vi "Launch Mission Actor.vi"(11 "RDS Root Actor in":refnum<class "RDS Root Actor.lvclass">) -> (3 "RDS Root Actor out":refnum<class "RDS Root Actor.lvclass">)   [LabVIEW 2015, in "RDS Root Actor.lvlib" / "RDS Root Actor.lvclass"]
uses:
  RDS Root Actor.lvclass
  Libraries/RDS Framework/RDS Message ID.ctl
  RDS Mission Controller Actor/RDS Mission Controller Actor/RDS Mission Controller Actor.lvclass
  RDS Mission Controller Actor/RDS Mission Controller Actor/RDS Mission Controller Actor.lvclass/RDS Mission Controller Actor.ctl
  RDS Parent Actor/RDS Parent Actor/RDS Parent Actor.lvclass/RDS Parent Actor.ctl
  RDS Parent Actor/RDS Parent Actor/RDS Parent Actor.lvclass
  Libraries/RDS Child Messages/RDS Child Messages.lvlib
  Libraries/Configuration Library/RDS Configuration Library.lvlib
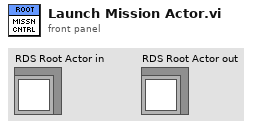
[diagram p1: front panel]
types:
  T1 = typedef "RDS Child Messages.lvlib/RDS Message ID.ctl" = enum16{"RDS Hello World", "String Message", "AIP_Status", "AIP_Command", "GPS_Data", "MCB_Command", "MCB_Status", "Compass_Data", "Depth_Data", "Battery_Data", "Contoller_State", "Set_Mag_Dev", "BTB_Shutdown", "State_Sample_Request", "State_Sample", "PID_Gains_Set", "Helm_Limiter_Set", "Helm_Heading_Command", "Helm_Steering_Command", "Helm_Status", "Controller_Message", "AIP_Set_Min_Depth", "Mission_Controller_State", "Mission_Upload", "Mission_Set_Op_and_Run", "Mission_Settings_Set"}
  T2 = typedef "RDS Configuration Library.lvlib/RDS Configuration.ctl" = cluster{"State Update Rate (Hz)":dbl, "Helm Rate (Hz)":dbl, "Helm Gains":T3, "Limiter":dbl, "Mission Controller Settings":T4, "Mag Dev":dbl}
  T3 = typedef "RDS Child Messages.lvlib/PID Gains Control.ctl" = cluster{"P (Kc)":sgl, "I (Ti)":sgl, "D (Td)":sgl}
  T4 = typedef "RDS Mission Controller Actor.lvlib/Mission Controller Settings.ctl" = cluster{"Waypoint Radius (m)":dbl}
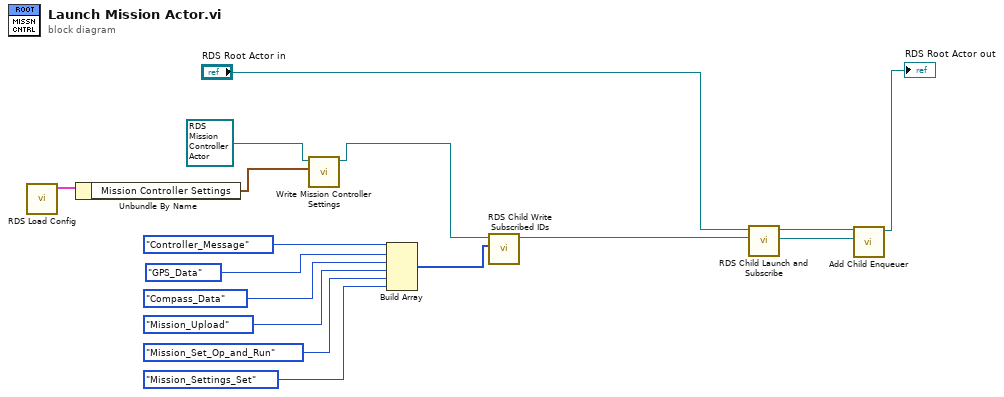
[diagram p0: block diagram]
diagram:
  n1 = call "RDS Load Config.vi"() -> ("RDS Config"=w7:T2)  [unwired: 11 in]
  n2 = Unbundle By Name(w7) -> ("Mission Controller Settings"=w6:T4)
  n3 = call "Write Mission Controller Settings.vi"("Mission Controller Settings"=w6, "RDS Mission Controller Actor in"=refnum<class "RDS Mission Controller Actor.lvclass"> refnum ("RDS Mission Controller Actor.lvlib:RDS Mission Controller Actor.lvclass")) -> ("RDS Mission Controller Actor out"=w8:refnum<class "RDS Mission Controller Actor.lvclass">)  [unwired: 8 in, 1 out]
  n4 = Build Array(RDS_Message_ID."Controller_Message" ("RDS Message"), RDS_Message_ID."GPS_Data" ("RDS Message"), RDS_Message_ID."Compass_Data" ("RDS Message"), RDS_Message_ID."Mission_Upload" ("RDS Message"), RDS_Message_ID."Mission_Set_Op_and_Run" ("RDS Message"), RDS_Message_ID."Mission_Settings_Set" ("RDS Message")) -> (w10:T1[])
  n5 = call "RDS Child Write Subscribed IDs.vi"("Subscribed IDs"=w10, "RDS Parent Actor in"=w8) -> ("RDS Parent Actor out"=w13:refnum<class "RDS Mission Controller Actor.lvclass">)  [unwired: 8 in, 1 out]
  n6 = call "RDS Child Launch and Subscribe.vi"("RDS Child in"=w13, "Caller Actor in"="RDS Root Actor in") -> ("Nested Actor's Enqueuer"=w15:refnum<class "Message Enqueuer.lvclass">, "Caller Actor Out"=w14:refnum<class "RDS Root Actor.lvclass">)  [unwired: 7 in, 1 out]
  n7 = call "Add Child Enqueuer.vi"("Nested Actor's Enqueuer"=w15, "RDS Root Actor in"=w14) -> ("RDS Root Actor out"=→"RDS Root Actor out":refnum<class "RDS Root Actor.lvclass">)  [unwired: 8 in, 1 out]
